vi "tearDown.vi"(8 "error in (no error)":errorcluster, 11 "reference in":refnum<class "BC Configuration.lvclass">) -> (0 "error out":errorcluster, 3 "reference out":refnum<class "BC Configuration.lvclass">)   [LabVIEW 2016, in "BC Configuration.lvclass"]
doc: "tearDown runs after the test method has completed. Use this method to clean up any operations or references that were opened by setUp or the test method. Unit tests should be independent of other unit tests so this VI should ensure that the next test can run in a 'clean' test environment."
uses:
  BC Configuration.lvclass
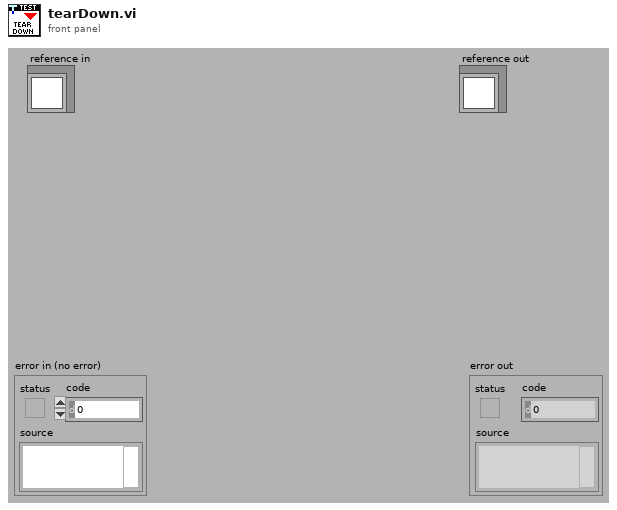
[diagram p1: front panel]
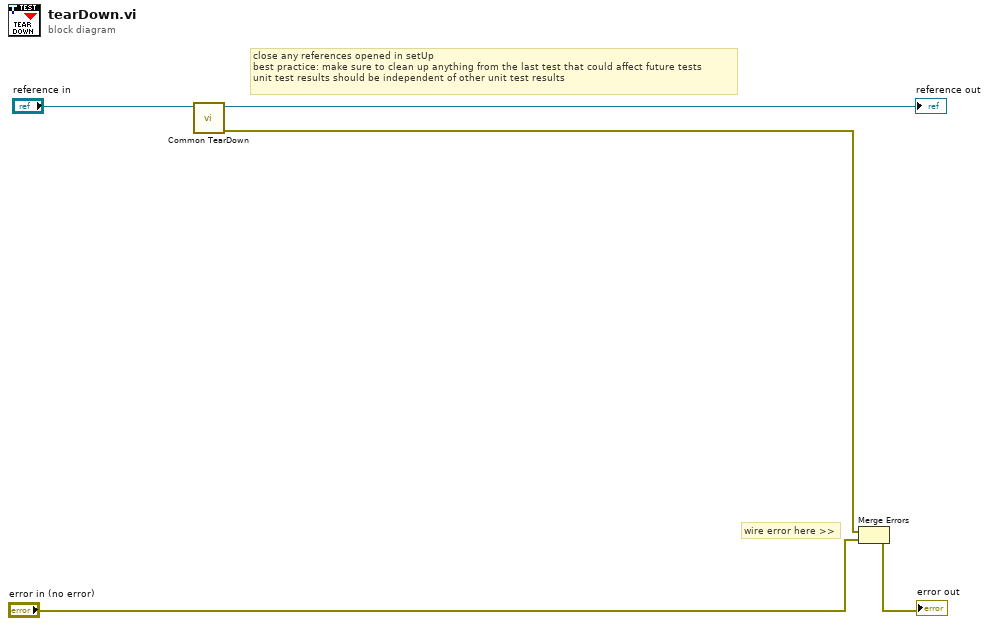
[diagram p0: block diagram]
diagram:
  # "wire error here >>"
  # "close any references opened in setUp\nbest practice: make sure to clean up anything from the last test that could affect future tests\nunit test results should be independent of other unit test results"
  n1 = call-dynamic "Common TearDown.vi"("1553 Test in"="reference in") -> ("error out"=w1:errorcluster, "1553 Test out"=→"reference out":refnum<class "BC Configuration.lvclass">)  [unwired: 9 in]
  n2 = Merge Errors(w1, "error in (no error)") -> (→"error out":errorcluster)
